vi "Convert directory new.vi"(8 "error in (no error)":errorcluster, 9 "directory out":path, 10 "directory in":path, 11 "DAQOrcaFlash in":refnum<class "DAQOrcaFlash.lvclass">) -> (0 "error out":errorcluster, 3 "DAQOrcaFlash out":refnum<class "DAQOrcaFlash.lvclass">)   [LabVIEW 2012, in "DAQOrcaFlash.lvclass"]
uses:
  DAQOrcaFlash.lvclass
  DAQOrcaFlash.lvclass/DAQOrcaFlash.ctl
  Lucid/LabVIEW/dependencies/classes/ImageCollection/ImageCollection.lvclass
  Lucid/LabVIEW/dependencies/classes/ImageCollection/storage_mode_enum.ctl
  Lucid/LabVIEW/dependencies/classes/Image/Image.lvclass
  Lucid/LabVIEW/dependencies/classes/Image/storage_mode.ctl
  Lucid/LabVIEW/dependencies/classes/ImageCollection/add_mode_enum.ctl
panel:
  in  "use tiff format? (F)":bool
  out "filename":string
  out "progress bar":sgl(slide) scale=0.0..1.0
  out "Files written to":path
  out "x+y":sgl
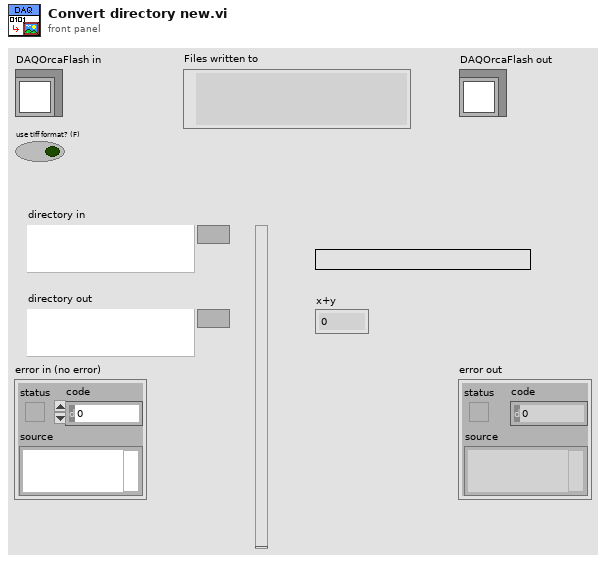
[diagram p1: front panel]
types:
  T1 = typedef "ImageCollection.lvclass/storage_mode_enum.ctl" = enum16{"RAM", "single files", "multipage TIFF (read-only)"}
  T2 = typedef "ImageCollection.lvclass/add_mode_enum.ctl" = enum16{"reference", "copy"}
  T3 = typedef "Image.lvclass/storage_mode.ctl" = enum16{"RAM", "disk"}
  T4 = typedef "Image Type" = u32
  T5 = typedef "IMAQ Image.ctl" = refnum<image>
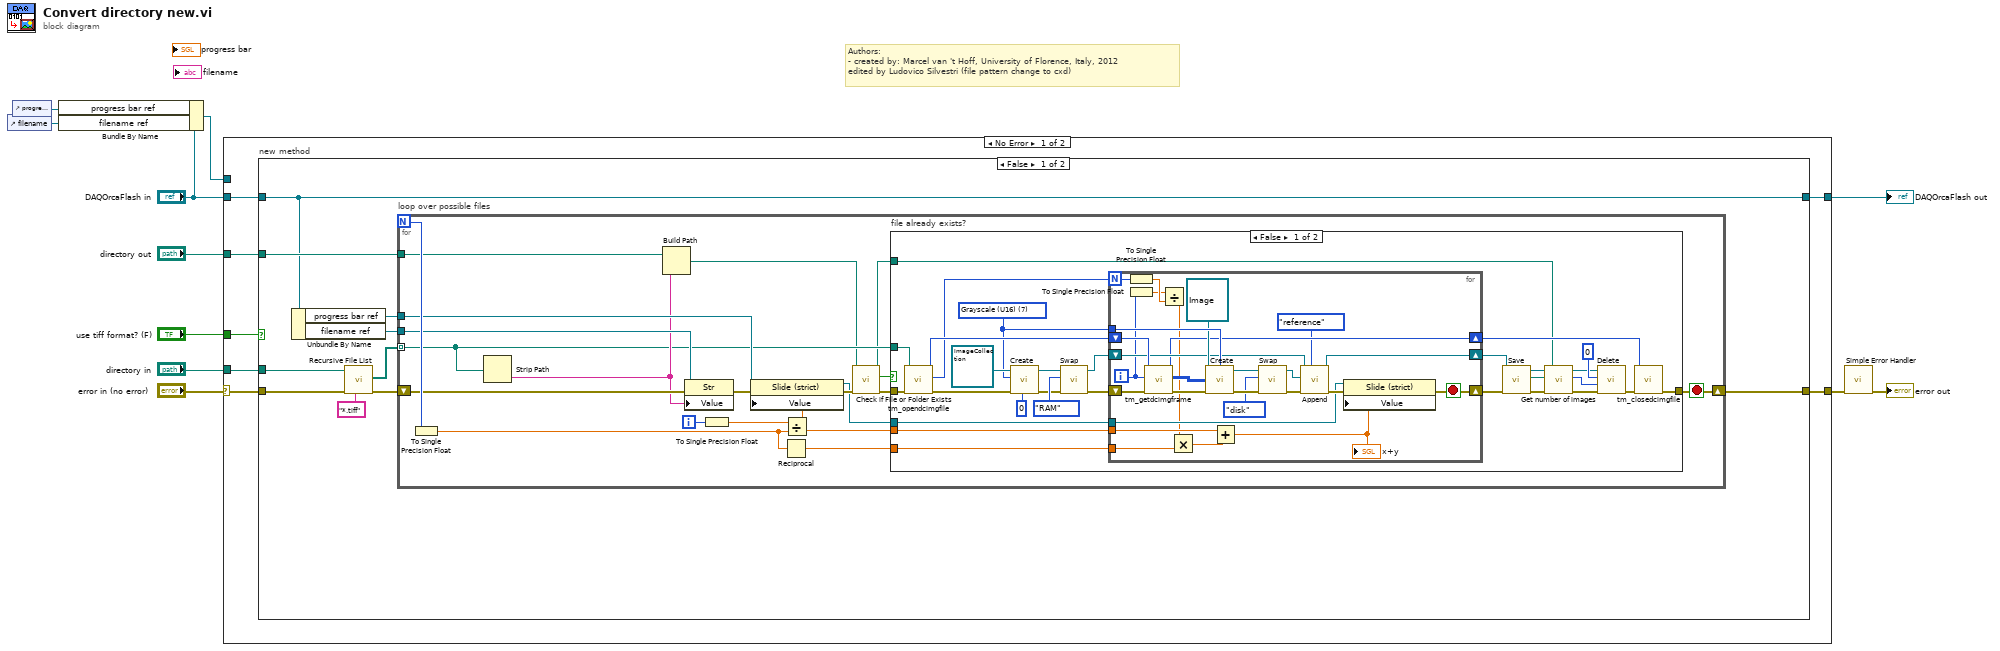
[diagram p0: block diagram]
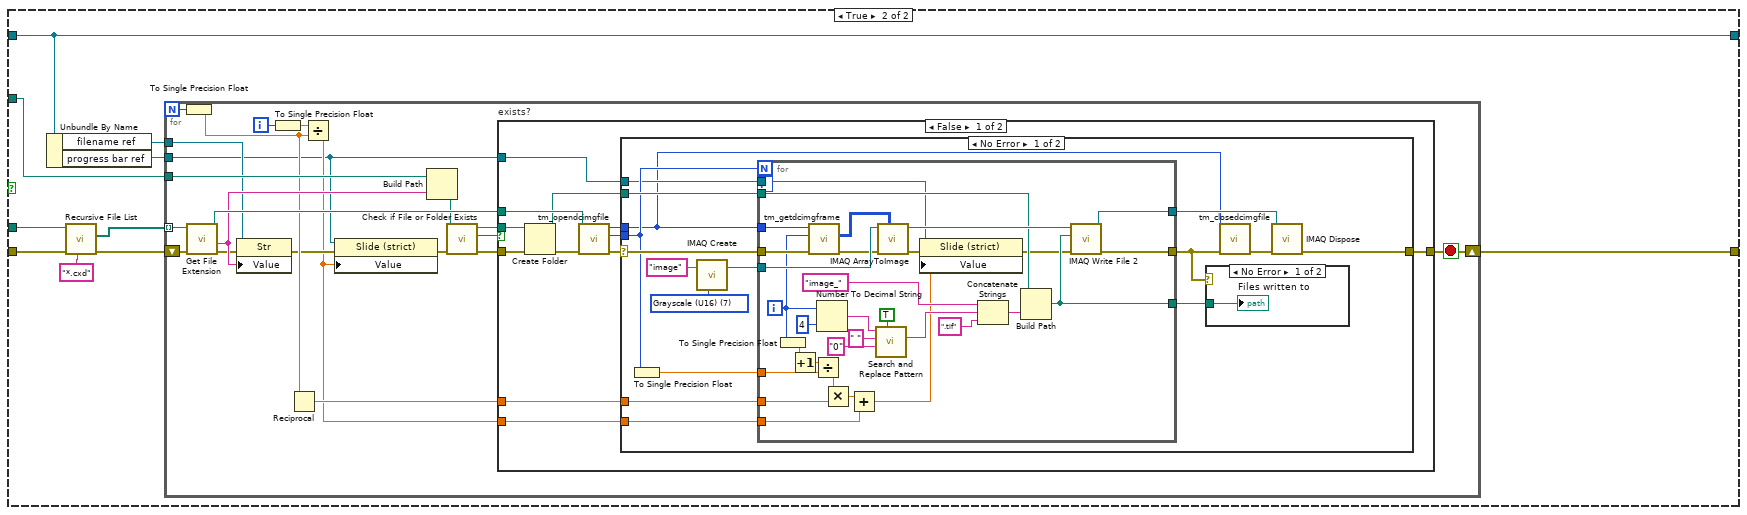
[diagram p3: hidden frame]
diagram:
  # "Authors: \n- created by: Marcel van 't Hoff, University of Florence, Italy, 2012\nedited by Ludovico Silvestri (file pattern change to cxd)"
  n1 = control-ref of="filename"() -> (w8:refnum<vi>)
  n2 = control-ref of="progress bar"() -> (w9:refnum<vi>)
  n3 = Bundle By Name(cluster="DAQOrcaFlash in", "progress bar ref"=w9, "filename ref"=w8) -> (w6:refnum<class "DAQOrcaFlash.lvclass">)
  n4 = case shown="No Error" "error in (no error)" {
    selector: "error in (no error)" -> [w17 w199]
    tunnel: [w14 w199] -> w7
    tunnel: [w13 w198] -> w3
    tunnel: "DAQOrcaFlash in" -> [w16 w198]
    tunnel: "directory in" -> [w18 _]
    tunnel: "directory out" -> [w15 _]
    tunnel: w6 -> [_ _]
    tunnel: "use tiff format? (F)" -> [w12 _]
    frame No Error {
      n5 = case "new method" shown="False" w12 {
        tunnel: w18 -> [w28 w112]
        tunnel: w17 -> [w27 w110]
        tunnel: w16 -> [w19 w107]
        tunnel: w15 -> [w21 w108]
        tunnel: [w20 w114] -> w14
        tunnel: [w19 w107] -> w13
        frame False {
          n6 = Unbundle By Name(w19) -> ("progress bar ref"=w23:refnum<vi>, "filename ref"=w22:refnum<vi>)
          n7 = call <vilib>:"Recursive File List.vi"("pattern"="*.tiff", "error in (no error)"=w27, "Folder Path"=w28) -> ("error out"=w24:errorcluster, "All Files in Dir"=w25:path[])  [unwired: 4 in, 3 out]
          n8 = for "loop over possible files" {
            N -> [w48]
            tunnel: w25 -> [w38] mode=indexing
            shift-right: [w39] -> w20
            shift-left: w24 -> [w45]
            tunnel: w23 -> [w46]
            tunnel: w22 -> [w44]
            tunnel: w21 -> [w43]
            i -> [w47]
            stop <- w39 stop-if-true
            n9 = To Single Precision Float(number=w48) -> (single precision float=w30:sgl)
            n10 = Strip Path(path=w38) -> (name=w42:string)  [unwired: 1 out]
            n11 = Build Path(base path=w43, name or relative path=w42) -> (appended path=w37:path)
            n12 = property class="Str"(reference=w44, error in=w45, "Value"=w42) -> (error out=w40:errorcluster)  [unwired: 1 out]
            n13 = To Single Precision Float(number=w47) -> (single precision float=w41:sgl)
            n14 = Reciprocal(x=w30) -> (1/x=w29:sgl)
            n15 = Divide(x=w41, y=w30) -> (x/y=w32:sgl)
            n16 = property class="Slide (strict)"(reference=w46, error in=w40, "Value"=w32) -> (reference out=w31:refnum<vi>, error out=w35:errorcluster)
            n17 = call <vilib>:"Check if File or Folder Exists.vi"("error in (no error)"=w35, "path"=w37) -> ("error out"=w34:errorcluster, "file or folder exists?"=w33:bool, "dup path"=w36:path)  [unwired: 7 in]
            n18 = case "file already exists?" shown="False" w33 {
              tunnel: [w60 w104] -> w39
              tunnel: w38 -> [w59 _]
              tunnel: w36 -> [w58 _]
              tunnel: w34 -> [w57 w104]
              tunnel: w32 -> [w56 _]
              tunnel: w31 -> [w55 _]
              tunnel: w29 -> [w54 _]
              frame False {
                w73 = T4 7 items=["Grayscale (U8)", "Grayscale (I16)", "Grayscale (SGL)", "Complex (CSG)", "RGB (U32)", "HSL (U32)", "RGB (U64)", "Grayscale (U16)"] ("Image Type")
                n19 = call <userlib>:"tm_opendcimgfile.vi"("error in (no error)"=w57, "Path"=w59) -> ("error out"=w75:errorcluster, "Total Frames"=w63:i32, "File Handle"=w74:u32)  [unwired: 7 in]
                n20 = call-dynamic "Create.vi"("size"=0, "error in (no error)"=w75, "Image Type"=w73, "ImageCollection in"=refnum<class "ImageCollection.lvclass"> refnum) -> ("error out"=w50:errorcluster, "ImageCollection out"=w53:refnum<class "ImageCollection.lvclass">)  [unwired: 6 in]
                n21 = call-dynamic "Swap.vi"("error in (no error)"=w50, "target storage mode"=storage_mode_enum."RAM" ("type"), "ImageCollection in"=w53) -> ("error out"=w49:errorcluster, "ImageCollection out"=w52:refnum<class "ImageCollection.lvclass">)  [unwired: 6 in, 1 out]
                n22 = for {
                  N: w63 -> [w89]
                  shift-right: [w83] -> w71
                  shift-left: w49 -> [w102]
                  tunnel: w73 -> [w99]
                  shift-right: [w96] -> w70
                  shift-left: w52 -> [w97]
                  shift-right: [w95] -> w61
                  shift-left: w74 -> [w103]
                  tunnel: w56 -> [w85]
                  tunnel: w55 -> [w81]
                  tunnel: w54 -> [w80]
                  i -> [w86]
                  stop <- w83 stop-if-true
                  n23 = To Single Precision Float(number=w89) -> (single precision float=w88:sgl)
                  n24 = To Single Precision Float(number=w86) -> (single precision float=w87:sgl)
                  n25 = call <userlib>:"tm_getdcimgframe.vi"("error in (no error)"=w102, "Frame Index"=w86, "File Handle in"=w103) -> ("error out"=w100:errorcluster, "Data"=w101:u16[][], "File Handle out"=w95:u32)  [unwired: 5 in, 1 out]
                  n26 = Divide(x=w87, y=w88) -> (x/y=w78:sgl)
                  n27 = Multiply(x=w78, y=w80) -> (x*y=w79:sgl)
                  n28 = call-dynamic "Create.vi"("Image in"=refnum<class "Image.lvclass"> refnum, "Image Type"=w99, "Image Pixels (U16)"=w101, "error in (no error)"=w100) -> ("Image out"=w94:refnum<class "Image.lvclass">, "error out"=w92:errorcluster)  [unwired: 10 in]
                  n29 = Add(x=w85, y=w79) -> (x+y=w82:sgl)
                  "x+y" <- w82
                  n30 = call-dynamic "Swap.vi"("error in (no error)"=w92, "storage type target"=storage_mode."disk" ("storage type"), "Image in"=w94) -> ("error out"=w91:errorcluster, "Image out"=w93:refnum<class "Image.lvclass">)  [unwired: 6 in, 1 out]
                  n31 = call-dynamic "Append.vi"("add mode (copy)"=add_mode_enum."reference", "error in (no error)"=w91, "Image.lvclass"=w93, "ImageCollection in"=w97) -> ("error out"=w84:errorcluster, "ImageCollection out"=w96:refnum<class "ImageCollection.lvclass">)  [unwired: 5 in, 1 out]
                  n32 = property class="Slide (strict)"(reference=w81, error in=w84, "Value"=w82) -> (error out=w83:errorcluster)  [unwired: 1 out]
                }
                n33 = call-dynamic "Save.vi"("error in (no error)"=w71, "path"=w58, "ImageCollection in"=w70) -> ("error out"=w66:errorcluster, "ImageCollection out"=w68:refnum<class "ImageCollection.lvclass">)  [unwired: 7 in]
                n34 = call-dynamic "Get number of images.vi"("error in (no error)"=w66, "ImageCollection in"=w68) -> ("error out"=w65:errorcluster, "size"=w64:i32, "ImageCollection out"=w67:refnum<class "ImageCollection.lvclass">)  [unwired: 7 in]
                n35 = call-dynamic "Delete.vi"("error in (no error)"=w65, "range"=w64, "start index"=0, "ImageCollection in"=w67) -> ("error out"=w62:errorcluster)  [unwired: 6 in, 1 out]
                n36 = call <userlib>:"tm_closedcimgfile.vi"("error in (no error)"=w62, "File Handle"=w61) -> ("error out"=w60:errorcluster)  [unwired: 9 in]
              }
              frame True {
              }
            }
          }
        }
        frame True {
          n37 = Unbundle By Name(w107) -> ("filename ref"=w106:refnum<vi>, "progress bar ref"=w105:refnum<vi>)
          n38 = call <vilib>:"Recursive File List.vi"("pattern"="*.cxd", "error in (no error)"=w110, "Folder Path"=w112) -> ("error out"=w109:errorcluster, "All Files in Dir"=w111:path[])  [unwired: 4 in, 3 out]
          n39 = for {
            N -> [w124]
            tunnel: w111 -> [w133] mode=indexing
            shift-right: [w128] -> w114
            shift-left: w109 -> [w134]
            tunnel: w108 -> [w135]
            tunnel: w106 -> [w125]
            tunnel: w105 -> [w117]
            i -> [w123]
            stop <- w128 stop-if-true
            n40 = To Single Precision Float(number=w124) -> (single precision float=w121:sgl)
            n41 = call <vilib>:"Get File Extension.vi"("error in (no error)"=w134, "file"=w133) -> ("error out"=w126:errorcluster, "filename without extension"=w127:string, "dup file"=w132:path)  [unwired: 6 in, 1 out]
            n42 = property class="Str"(reference=w125, error in=w126, "Value"=w127) -> (error out=w120:errorcluster)  [unwired: 1 out]
            n43 = To Single Precision Float(number=w123) -> (single precision float=w122:sgl)
            n44 = Reciprocal(x=w121) -> (1/x=w119:sgl)
            n45 = Divide(x=w122, y=w121) -> (x/y=w118:sgl)
            n46 = property class="Slide (strict)"(reference=w117, error in=w120, "Value"=w118) -> (error out=w115:errorcluster)  [unwired: 1 out]
            n47 = Build Path(base path=w135, name or relative path=w127) -> (appended path=w116:path)
            n48 = call <vilib>:"Check if File or Folder Exists.vi"("error in (no error)"=w115, "path"=w116) -> ("error out"=w130:errorcluster, "file or folder exists?"=w129:bool, "dup path"=w131:path)  [unwired: 7 in]
            n49 = case "exists?" shown="False" w129 {
              tunnel: [w144 w197] -> w128
              tunnel: w132 -> [w143 _]
              tunnel: w131 -> [w139 _]
              tunnel: w130 -> [w137 w197]
              tunnel: w119 -> [w142 _]
              tunnel: w118 -> [w141 _]
              tunnel: w117 -> [w140 _]
              frame False {
                n50 = Create Folder(path (use dialog)=w139, error in=w137) -> (created path=w138:path, error out=w136:errorcluster)  [unwired: 1 in, 1 out]
                n51 = call <userlib>:"tm_opendcimgfile.vi"("error in (no error)"=w136, "Path"=w143) -> ("error out"=w145:errorcluster, "Total Frames"=w147:i32, "File Handle"=w146:u32)  [unwired: 7 in]
                n52 = case shown="No Error" w145 {
                  selector: w145 -> [w163 w196]
                  tunnel: w146 -> [w148 _]
                  tunnel: [w156 w196] -> w144
                  tunnel: w147 -> [w153 _]
                  tunnel: w138 -> [w158 _]
                  tunnel: w142 -> [w151 _]
                  tunnel: w141 -> [w150 _]
                  tunnel: w140 -> [w149 _]
                  frame No Error {
                    w161 = T4 7 items=["Grayscale (U8)", "Grayscale (I16)", "Grayscale (SGL)", "Complex (CSG)", "RGB (U32)", "HSL (U32)", "RGB (U64)", "Grayscale (U16)"] ("Image Type")
                    n53 = To Single Precision Float(number=w153) -> (single precision float=w152:sgl)
                    n54 = call "IMAQ Create"("Image Name"="image", "Image Type"=w161) -> ("New Image"=w160:T5)  [unwired: 3 in, 1 out]
                    n55 = for {
                      N: w153 -> [_]
                      tunnel: w160 -> [w193]
                      tunnel: w158 -> [w179]
                      tunnel: [w178] -> w155
                      tunnel: [w177] -> w154
                      tunnel: w152 -> [w176]
                      tunnel: w151 -> [w173]
                      tunnel: w150 -> [w170]
                      tunnel: w149 -> [w166]
                      tunnel: w163 -> [w194]
                      tunnel: [w180] -> w159
                      tunnel: w148 -> [w195]
                      workers-P: _ -> [_]
                      i -> [w175]
                      n56 = To Single Precision Float(number=w175) -> (single precision float=w174:sgl)
                      n57 = Increment(x=w174) -> (x+1=w165:sgl)
                      n58 = call <userlib>:"tm_getdcimgframe.vi"("error in (no error)"=w194, "Frame Index"=w175, "File Handle in"=w195) -> ("error out"=w191:errorcluster, "Data"=w181:u16[][])  [unwired: 5 in, 2 out]
                      n59 = Divide(x=w165, y=w176) -> (x/y=w172:sgl)
                      n60 = Number To Decimal String(number=w175, width (-)=i16 4) -> (decimal integer string=w188:string)
                      n61 = Multiply(x=w172, y=w173) -> (x*y=w171:sgl)
                      n62 = Add(x=w171, y=w170) -> (x+y=w169:sgl)
                      n63 = call <vilib>:"Search and Replace Pattern.vi"("string"=w188, "regular expression (\"\")"=" " ("regular expression (\"\")"), "replace string (\"\")"="0" ("replace string (\"\")"), "replace all? (F)"=TRUE) -> ("result string"=w184:string)  [unwired: 1 in, 1 out]
                      n64 = call "IMAQ ArrayToImage"("Image Pixels (U16)"=w181, "error in (no error)"=w191, "Image"=w193) -> ("error out"=w168:errorcluster, "Image Out"=w192:T5)  [unwired: 7 in]
                      n65 = property class="Slide (strict)"(reference=w166, error in=w168, "Value"=w169) -> (error out=w167:errorcluster)  [unwired: 1 out]
                      n66 = Concatenate Strings("image_", w184, ".tif" ("regular expression (\"\")")) -> (w183:string)
                      n67 = Build Path(base path=w179, name or relative path=w183) -> (appended path=w177:path)
                      n68 = call-poly "IMAQ Write File 2"("error in (no error)"=w167, "File Path"=w177, "Image"=w192) -> ("error out"=w180:errorcluster, "Image Out (duplicate)"=w178:T5)  [unwired: 7 in]
                    }
                    n69 = case shown="No Error" w159 {
                      tunnel: w154 -> [w164 _]
                      frame No Error {
                        "Files written to" <- w164
                      }
                      frame Error {
                      }
                    }
                    n70 = call <userlib>:"tm_closedcimgfile.vi"("error in (no error)"=w159, "File Handle"=w148) -> ("error out"=w157:errorcluster)  [unwired: 9 in]
                    n71 = call "IMAQ Dispose"("Image"=w155, "error in (no error)"=w157) -> ("error out"=w156:errorcluster)  [unwired: 4 in]
                  }
                  frame Error {
                  }
                }
              }
              frame True {
              }
            }
          }
        }
      }
    }
    frame Error {
    }
  }
  "DAQOrcaFlash out" <- w3
  n72 = call <vilib>:"Simple Error Handler.vi"("error in (no error)"=w7) -> ("error out"=→"error out":errorcluster)  [unwired: 4 in, 4 out]
